vi "GetSurfacePixels.vi"(8 "No Error":errorcluster, 11 "Surface [SDL_Surface *]":i64) -> (0 "error out":errorcluster, 2 "Surface Info":T3 {"flag" items=["SDL_SURFACE_PREALLOCATED"=1, "SDL_SURFACE_LOCK_NEEDED"=2, "SDL_SURFACE_LOCKED"=4, "SDL_SURFACE_SIMD_ALIGNED"=8]}, 3 "Pixels":u8[](array[numeric]) format="%.0x")   [LabVIEW 2026, in "SDL3.lvlib" / "Surface.lvlib"]
doc: "<B>Summary</B>\nRead surface pixels."
uses:
  Surface.lvlib
  SurfaceFlags--ring.ctl
  Pixels/PixelFormat--enum.ctl
  LV-Utilities/IsNULL.vi
  Pixels/U32ToPixelFormatEnum.vi
  Error/GetError-AnyThread.vi
  LV-Utilities/PointerSize.vi
  <vilib>/Utility/error.llb/Error Cluster From Error Code.vi
  LV-Utilities/LV-Utilities.lvlib
  Pixels/Pixels.lvlib
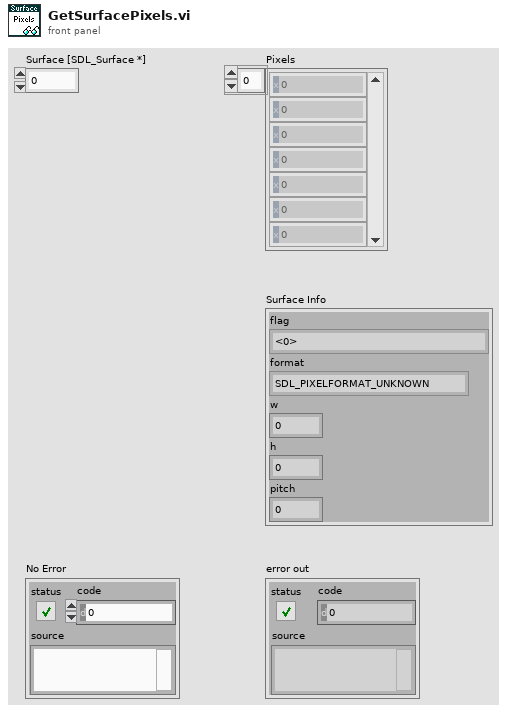
[diagram p1: front panel]
types:
  T1 = typedef "SDL3.lvlib/Surface.lvlib/SurfaceFlags--ring.ctl" = u32
  T2 = typedef "SDL3.lvlib/Pixels.lvlib/PixelFormat--enum.ctl" = enum32{"SDL_PIXELFORMAT_UNKNOWN", "SDL_PIXELFORMAT_INDEX1LSB", "SDL_PIXELFORMAT_INDEX1MSB", "SDL_PIXELFORMAT_INDEX2LSB", "SDL_PIXELFORMAT_INDEX2MSB", "SDL_PIXELFORMAT_INDEX4LSB", "SDL_PIXELFORMAT_INDEX4MSB", "SDL_PIXELFORMAT_INDEX8", "SDL_PIXELFORMAT_RGB332", "SDL_PIXELFORMAT_XRGB4444", "SDL_PIXELFORMAT_XBGR4444", "SDL_PIXELFORMAT_XRGB1555", "SDL_PIXELFORMAT_XBGR1555", "SDL_PIXELFORMAT_ARGB4444", "SDL_PIXELFORMAT_RGBA4444", "SDL_PIXELFORMAT_ABGR4444", "SDL_PIXELFORMAT_BGRA4444", "SDL_PIXELFORMAT_ARGB1555", "SDL_PIXELFORMAT_RGBA5551", "SDL_PIXELFORMAT_ABGR1555", "SDL_PIXELFORMAT_BGRA5551", "SDL_PIXELFORMAT_RGB565", "SDL_PIXELFORMAT_BGR565", "SDL_PIXELFORMAT_RGB24", "SDL_PIXELFORMAT_BGR24", "SDL_PIXELFORMAT_XRGB8888", "SDL_PIXELFORMAT_RGBX8888", "SDL_PIXELFORMAT_XBGR8888", "SDL_PIXELFORMAT_BGRX8888", "SDL_PIXELFORMAT_ARGB8888", "SDL_PIXELFORMAT_RGBA8888", "SDL_PIXELFORMAT_ABGR8888", "SDL_PIXELFORMAT_BGRA8888", "SDL_PIXELFORMAT_XRGB2101010", "SDL_PIXELFORMAT_XBGR2101010", "SDL_PIXELFORMAT_ARGB2101010", "SDL_PIXELFORMAT_ABGR2101010", "SDL_PIXELFORMAT_RGB48", "SDL_PIXELFORMAT_BGR48", "SDL_PIXELFORMAT_RGBA64", "SDL_PIXELFORMAT_ARGB64", "SDL_PIXELFORMAT_BGRA64", "SDL_PIXELFORMAT_ABGR64", "SDL_PIXELFORMAT_RGB48_FLOAT", "SDL_PIXELFORMAT_BGR48_FLOAT", "SDL_PIXELFORMAT_RGBA64_FLOAT", "SDL_PIXELFORMAT_ARGB64_FLOAT", "SDL_PIXELFORMAT_BGRA64_FLOAT", "SDL_PIXELFORMAT_ABGR64_FLOAT", "SDL_PIXELFORMAT_RGB96_FLOAT", "SDL_PIXELFORMAT_BGR96_FLOAT", "SDL_PIXELFORMAT_RGBA128_FLOAT", "SDL_PIXELFORMAT_ARGB128_FLOAT", "SDL_PIXELFORMAT_BGRA128_FLOAT", "SDL_PIXELFORMAT_ABGR128_FLOAT", "SDL_PIXELFORMAT_YV12", "SDL_PIXELFORMAT_IYUV", "SDL_PIXELFORMAT_YUY2", "SDL_PIXELFORMAT_UYVY", "SDL_PIXELFORMAT_YVYU", "SDL_PIXELFORMAT_NV12", "SDL_PIXELFORMAT_NV21", "SDL_PIXELFORMAT_P010", "SDL_PIXELFORMAT_EXTERNAL_OES"}
  T3 = cluster{"flag":T1, "format":T2, "w":i32, "h":i32, "pitch":i32}
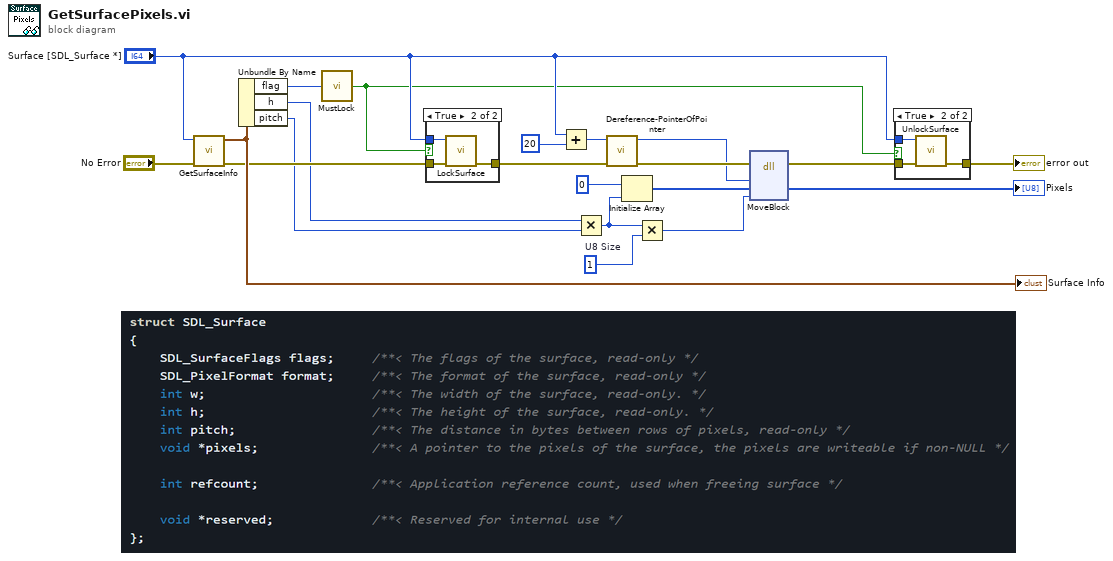
[diagram p0: block diagram]
diagram:
  w12 = 1  # U8 Size
  n1 = call "GetSurfaceInfo.vi"("No Error"="No Error", "Surface [SDL_Surface *]"="Surface [SDL_Surface *]") -> ("error out"=w10:errorcluster, "Surface Info"=w17:T3)  [unwired: 8 in]
  "Surface Info" <- w17
  n2 = Unbundle By Name(w17) -> ("flag"=w7:T1, "h"=w6:i32, "pitch"=w5:i32)
  n3 = call "MustLock.vi"("SurfaceFlags"=w7) -> ("Must Lock?"=w8:bool)
  n4 = case shown="True" w8 {
    tunnel: w10 -> [w22 w25]
    tunnel: [w22 w24] -> w4
    tunnel: "Surface [SDL_Surface *]" -> [_ w23]
    frame False {
    }
    frame True {
      n5 = call "LockSurface.vi"("No Error"=w25, "Surface [SDL_Surface *]"=w23) -> ("error out"=w24:errorcluster)  [unwired: 9 in]
    }
  }
  n6 = Add(x="Surface [SDL_Surface *]", y=i64 20) -> (x+y=w2:i64)
  n7 = Multiply(x=w6, y=w5) -> (x*y=w11:i32)
  n8 = call "Dereference-PointerOfPointer.vi"("No Error"=w4, "Ptr of Ptr [void **]"=w2) -> ("error out"=w3:errorcluster, "Ptr [void *]"=w1:i64)  [unwired: 8 in]
  n9 = Initialize Array(u8 0, w11) -> (w15:u8[])
  n10 = Multiply(x=w11, y=w12) -> (x*y=w13:i32)
  n11 = dll-call lib="LabVIEW" fn="MoveBlock"(error in=w3, "Address"=w1, "Destination"=w15, "Size"=w13) -> (error out=w9:errorcluster, "Destination"=→"Pixels":u8[])  [unwired: 5 in, 1 out]
  n12 = case shown="True" w8 {
    tunnel: w9 -> [w26 w29]
    tunnel: [w26 w28] -> w20
    tunnel: "Surface [SDL_Surface *]" -> [_ w27]
    frame False {
    }
    frame True {
      n13 = call "UnlockSurface.vi"("No Error"=w29, "Surface [SDL_Surface *]"=w27) -> ("error out"=w28:errorcluster)  [unwired: 9 in]
    }
  }
  "error out" <- w20
